vi "MHM Get Cal Param.vi"(8 "error in (no error)":errorcluster, 10 "ulParam":u32, 11 "ulMHMHandle":u32) -> (0 "error out":errorcluster, 2 "plData":i32, 3 "function return":u32)   [LabVIEW 2017, in "MHM_1SL_interface.lvlib"]
uses:
  MHM_1SL_interface.lvlib
  SSI_Tool/DUT_Interface/lv_interface/lib/MHM_1SL_interface.dll
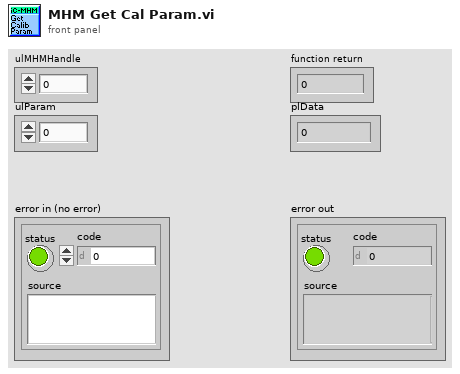
[diagram p1: front panel]
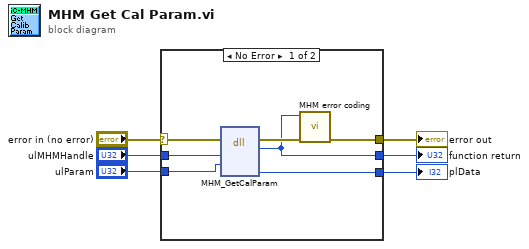
[diagram p0: block diagram]
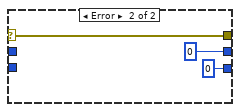
[diagram p2: hidden frame]
diagram:
  n1 = case shown="No Error" "error in (no error)" {
    selector: "error in (no error)" -> [w13 w16]
    tunnel: "ulMHMHandle" -> [w12 _]
    tunnel: [w10 w16] -> w4
    tunnel: [w9 u32 0] -> w3
    tunnel: "ulParam" -> [w8 _]
    tunnel: [w7 0 ("plData")] -> w1
    frame No Error {
      n2 = dll-call lib="C:/workspace/project/scancon/sw/SSI_Tool/DUT_Interface/lv_interface/lib/MHM_1SL_interface.dll" fn="MHM_GetCalParam"(error in=w13, "ulMHMHandle"=w12, "ulParam"=w8) -> (error out=w11:errorcluster, "return type"=w9:u32, "plData"=w7:i32)  [unwired: 5 in, 1 out]
      n3 = call "MHM error coding.vi"("error in (no error)"=w11, "function return in"=w9) -> ("error out"=w10:errorcluster)  [unwired: 9 in]
    }
    frame Error {
    }
  }
  "function return" <- w3
  "error out" <- w4
  "plData" <- w1
